vi "Simulation - Cascade and Feedforward Surge Tank Level.vi"() -> ()   [LabVIEW 2023]
doc: "This example demonstrates a process simulation for a surge tank level with cascade and feedforward controller. The process has added noise, valve deadband, lag, and deadtime. A inflow adjusts the level of the tank. The Surge Profile allow you to apply an specific variation of flow."
uses:
  <vilib>/addons/control/pid/pid.llb/PID Lead-Lag (DBL).vi
  <vilib>/addons/control/pid/pid.llb/PID (DBL).vi
  <vilib>/addons/control/pid/NI_PID_pid.lvlib
panel:
  in  "Tab Control":enum32{"Introduction", "Profile", "Diagram"}(tab)
  out "Inflow Profile Graph":cluster{dbl, dbl}[](graph)
  in  "Apply Inflow Profile":bool=TRUE
  in  "Constant Flow (%)":dbl=40.0
  in  "Inflow Profile":cluster{"time (s)":dbl, "setpoint":dbl}[](array[cluster])=[{"time (s)"=0.0, "setpoint"=40.0}, {"time (s)"=10.0, "setpoint"=40.0}, {"time (s)"=10.0, "setpoint"=60.0}, {"time (s)"=20.0, "setpoint"=60.0}]
  out "FT-2 Valve":dbl(knob)=84.28886007445381 scale=0.0..100.0
  out "control valve":dbl=86.66603993277398 format="%.2f"
  out "Valve":bool
  out "Pump":bool=TRUE
  out "Surge Tank":dbl(slide)=49.279730305904245 scale=0.0..100.0 scale format="%.2f"
  out "FT-2":dbl(knob)=84.28886007445381 scale=0.0..100.0
  out "LT 1":dbl=49.279730305904245
  in  "Feedforward\nLag Time (min)":dbl(slide)=0.9102981779915218 scale=0.01..10.0
  out "SP2:":dbl(slide)=140.87020302841148 min=0.0 max=0.0 scale=0.0..100.0
  out "MV2:":dbl(slide)=86.66603993277398 scale=0.0..100.0
  out "PV2:":dbl(slide)=83.29836846682039 scale=0.0..100.0
  out "SP1:":dbl(slide)=40.87020302841148 min=0.0 max=0.0 scale=0.0..100.0
  out "MV1:":dbl(slide)=100.0 scale=-100.0..100.0
  out "PV1:":dbl(slide)=50.762476114859936 scale=0.0..100.0
  in  "PID parameters (FC)":T1={"Kc"=1.0, "Ti (min)"=0.08, "Td (min)"=0.0} {"Td (min)" format="%#.6f"; "Ti (min)" format="%#.4f"; "Kc" format="%#.4f"}
  in  "PID parameters (LC)":T1={"Kc"=-20.0, "Ti (min)"=0.1, "Td (min)"=0.0} {"Td (min)" format="%#.6f"; "Ti (min)" format="%#.4f"; "Kc" format="%#.4f"}
  in  "Stop":bool
  out "Process Chart":T2(graph)={"Constant Flow (%)"=40.0, "Valve Deadband"=49.279730305904245, "output"=84.28886007445381}
  # "Level Controller (LC)"
  # "Flow Controller (FC)"
  # "Feedforward value defines the behavior of the Tank\nLg=1-> Outflow tracks Inflow\nLg=0.1-> Outflow tracks Level\nLg=0.01-> Level tracks Inflow"
  # "Reverse Action is obtained by using negative gain for Kc"
  # "Overview: This example demonstrates a process simulation for a surge tank level with cascade and feedforward controller.  A surge tank is used to absorb sudden rises of pressure. The Inflow Profile allows you to apply an specific surge flow variation.The tank model has added noise, valve deadband, lag, and deadtime.\nInstructions:\n1. Run the VI.\n2. Verify the setpoint profile being generated and the controller tracking its value.\n3. Go to the Diagram tab and see the animation of the process implemented. The Process Chart will show the signals to be used.\n4. Change the Feedforward Lag Time. You can see the following behavior:\na. Lg=1-> Output flow (outflow) tracks input flow (inflow) changes\nb. Lg=0.1-> Output flow tracks Level changes\nc. Lg=0.01-> Level tracks input flow changes\n5. Note that the Level Controller needs a Reverse Action on the controller. This is obtained by negating Kc.\n6. Click Stop to stop the VI."
  # "ISA Symbology: The diagram uses the ISA Symbology used for control"
  # "Level Controller (LC) or Flow Controller (FC) in a panel"
  # "Loop 1"
  # "Loop 2"
  # "Level Transmitter on the field"
  # "Flow Transmitter \non the field"
  # "FC"
  # "LT"
  # "1"
  # "FT"
  # "2"
  # "LC"
  # "Time (s)"
  # "Flow (%)"
  # "///"
  # "///"
  # "///"
  # "SP"
  # "///"
  # "///"
  # "1"
  # "SP"
  # "///"
  # "2"
  # "%"
  # "%"
  # "FC"
  # "FT"
  # "2"
  # "LT"
  # "1"
  # "+"
  # "+"
  # "S"
  # "Feedforward"
  # "T"
  # "id"
  # "LC"
  # "FT"
  # "1"
  # "%"
  # "%"
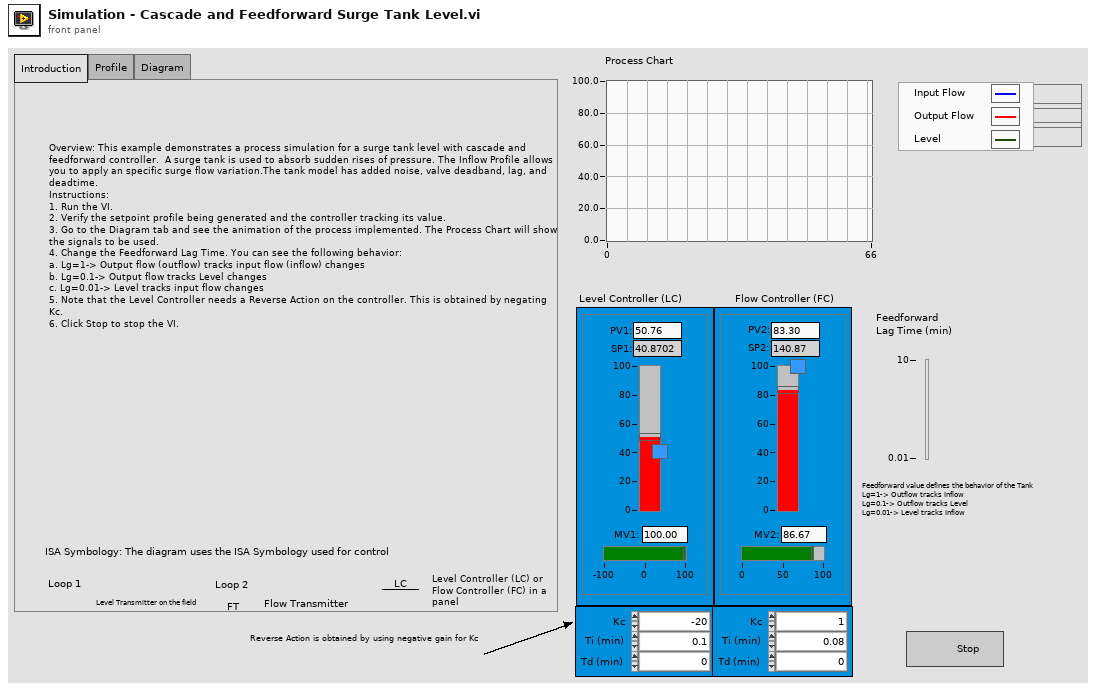
[diagram p1: front panel]
types:
  T1 = cluster{"Kc":dbl, "Ti (min)":dbl, "Td (min)":dbl}
  T2 = cluster{"Constant Flow (%)":dbl, "Valve Deadband":dbl, "output":dbl}
  T3 = cluster{"gain":dbl, "lag time (min)":dbl, "lead time (min)":dbl}
  T4 = cluster{"Constant Flow (%)":dbl, "output":dbl, "Valve Deadband":dbl}
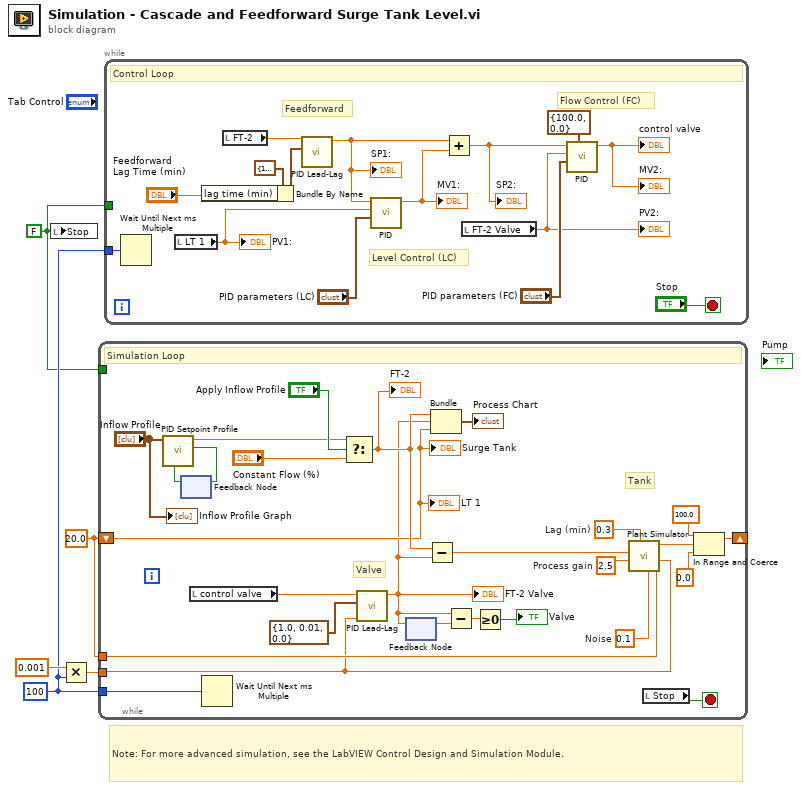
[diagram p0: block diagram]
diagram:
  w1 = FALSE ("Stop")
  w2 = 100
  w5 = 20.0 ("Valve Deadband")
  # "Note: For more advanced simulation, see the LabVIEW Control Design and Simulation Module."
  n1 = local write "Stop"(w1) -> ()
  n2 = Multiply(x=0.001, y=w2) -> (x*y=w3:dbl)
  n3 = while {
    shift-left: w5 -> [w13]
    shift-right: [w21] -> _
    tunnel: w5 -> [w20]
    tunnel: w3 -> [w12]
    tunnel: w2 -> [w11]
    tunnel: w1 -> [_]
    stop <- w30 stop-if-true
    w27 = 0.3  # Lag (min)
    w26 = 2.5  # Process gain
    w25 = 0.1  # Noise
    # "Tank"
    # "Valve"
    # "Simulation Loop"
    n4 = feedback #1() -> (w31:bool)  [unwired: 1 in]
    n5 = call <vilib>:"PID Setpoint Profile.vi"("reinitialize? (F)"=w31, "setpoint profile"="Inflow Profile") -> ("profile complete?"=w32:bool, "setpoint"=w15:dbl)  [unwired: 4 in, 2 out]
    n6 = feedback-in #1(w32) -> ()
    n7 = local read "control valve"() -> (w17:dbl)
    n8 = Wait Until Next ms Multiple(millisecond multiple=w11) -> ()  [unwired: 1 out]
    n9 = Select(t=w15, s="Apply Inflow Profile", f="Constant Flow (%)") -> (s? t:f=w16:dbl)
    "FT-2" <- w16
    n10 = call-poly <vilib>:"PID Lead-Lag.vi"("dt (s)"=w12, "tuning parameters"=T3 {"gain"=1.0, "lag time (min)"=0.01, "lead time (min)"=0.0}, "input"=w17) -> ("output"=w8:dbl)  [unwired: 5 in, 1 out]
    "FT-2 Valve" <- w8
    n11 = feedback-in #2(w8) -> ()
    n12 = feedback #2() -> (w9:dbl)  [unwired: 1 in]
    n13 = Subtract(x=w16, y=w8) -> (x-y=w19:dbl)
    n14 = Bundle("Constant Flow (%)"=w16, "output"=w8, "Valve Deadband"=w13) -> (→"Process Chart":T4)  [unwired: 1 in]
    n15 = Subtract(x=w8, y=w9) -> (x-y=w7:dbl)
    n16 = Greater Or Equal To 0?(x=w7) -> (x >= 0?=→"Valve":bool)
    n17 = call "Plant Simulator.vi"("Initial PV"=w20, "dt (s)"=w12, "Controller Noise (%)"=w25, "Lag (min)"=w27, "Process Gain"=w26, "Manipulated Variable (Output, %)"=w19) -> ("Process Variable (%)"=w24:dbl)  [unwired: 5 in]
    n18 = local read "Stop"() -> (w30:bool)
    n19 = In Range and Coerce(upper limit=100.0, x=w24, lower limit=0.0) -> (coerced(x)=w21:dbl)  [unwired: 1 out]
    "Surge Tank" <- w13
    "LT 1" <- w13
    "Inflow Profile Graph" <- "Inflow Profile"
  }
  n20 = while {
    tunnel: w2 -> [w33]
    tunnel: w1 -> [_]
    stop <- "Stop" stop-if-true
    # "Flow Control (FC)"
    # "Level Control (LC)"
    # "Feedforward"
    # "Control Loop"
    n21 = Wait Until Next ms Multiple(millisecond multiple=w33) -> ()  [unwired: 1 out]
    n22 = local read "LT 1"() -> (w38:dbl)
    "PV1:" <- w38
    n23 = Bundle By Name(cluster=T3 {"gain"=1.0, "lag time (min)"=0.01, "lead time (min)"=0.0} ("tuning parameters"), "lag time (min)"="Feedforward\nLag Time (min)") -> (w36:T3)
    n24 = local read "FT-2"() -> (w43:dbl)
    n25 = call-poly <vilib>:"PID Lead-Lag.vi"("tuning parameters"=w36, "input"=w43) -> ("output"=w39:dbl)  [unwired: 6 in, 1 out]
    "SP1:" <- w39
    n26 = call-poly <vilib>:"PID.vi"("PID gains"="PID parameters (LC)", "process variable"=w38, "setpoint"=w39) -> ("output"=w44:dbl)  [unwired: 7 in, 1 out]
    "MV1:" <- w44
    n27 = Add(x=w39, y=w44) -> (x+y=w40:dbl)
    "SP2:" <- w40
    n28 = local read "FT-2 Valve"() -> (w37:dbl)
    "PV2:" <- w37
    n29 = call-poly <vilib>:"PID.vi"("output range"=cluster{"output high":dbl, "output low":dbl} {"output high"=100.0, "output low"=0.0}, "PID gains"="PID parameters (FC)", "process variable"=w37, "setpoint"=w40) -> ("output"=→"control valve" →"MV2:":dbl)  [unwired: 6 in, 1 out]
  }
